vi "COM_get_data.vi"(8 "data":u8[](array[numeric]), 10 "baud rate (9600)":u32=115200 caption="波特率(115200)", 11 "VISA name":refnum<visa-resource-name>) -> (2 "data out":u8[](array[numeric]), 3 "return":i32)   [LabVIEW 2016]
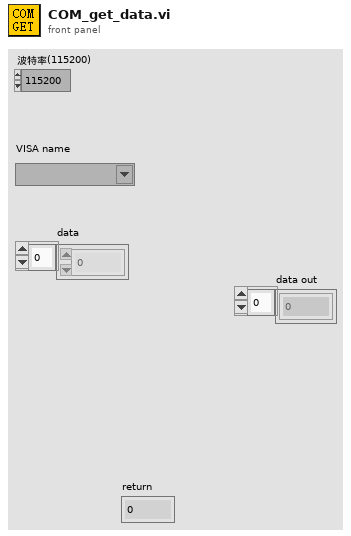
[diagram p1: front panel]
types:
  T1 = enum16{"initial", "write", "read", "release", "change"}
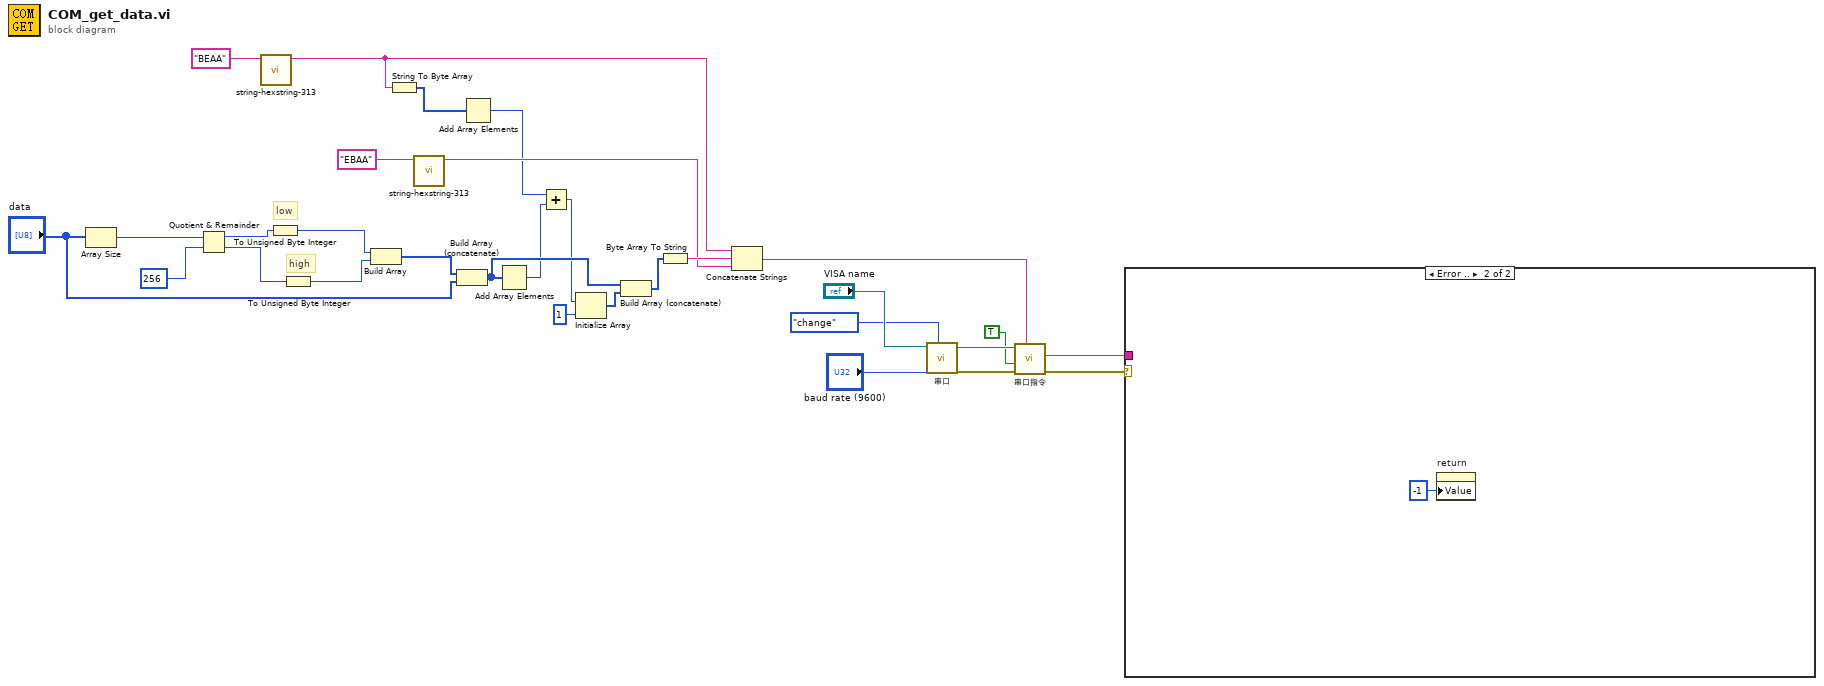
[diagram p0: block diagram]
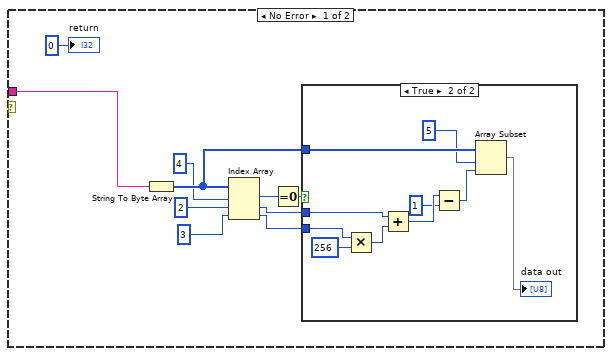
[diagram p2: hidden frame]
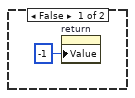
[diagram p3: hidden frame]
diagram:
  # "high"
  # "low"
  n1 = Array Size(array="data") -> (size(s)=w10:i32)
  n2 = Quotient & Remainder(x=w10, y=256) -> (x-y*floor(x/y)=w28:i32, floor(x/y)=w29:i32)
  n3 = call "string-hexstring-313.vi"("字符串"="BEAA") -> ("十六进制整型字符串"=w15:string)  [unwired: 10 in]
  n4 = To Unsigned Byte Integer(number=w28) -> (unsigned 8bit integer=w26:u8)
  n5 = To Unsigned Byte Integer(number=w29) -> (unsigned 8bit integer=w25:u8)
  n6 = Build Array(w26, w25) -> (w24:u8[])
  n7 = String To Byte Array(string=w15) -> (unsigned byte array=w14:u8[])
  n8 = call "string-hexstring-313.vi"("字符串"="EBAA") -> ("十六进制整型字符串"=w16:string)  [unwired: 10 in]
  n9 = Build Array (concatenate)(w24, "data") -> (w19:u8[])
  n10 = Add Array Elements(numeric array=w14) -> (sum=w13:u8)
  n11 = Add Array Elements(numeric array=w19) -> (sum=w12:u8)
  n12 = Add(x=w13, y=w12) -> (x+y=w11:u8)
  n13 = Initialize Array(w11, 1 ("dimension size")) -> (w20:u8[])
  n14 = Build Array (concatenate)(w19, w20) -> (w18:u8[])
  n15 = Byte Array To String(unsigned byte array=w18) -> (string=w22:string)
  n16 = Concatenate Strings(w15, w22, w16) -> (w4:string)
  n17 = call "串口.vi"("case"=T1."change", "baud rate (9600)"="baud rate (9600)", "VISA name"="VISA name") -> ("error out"=w5:errorcluster, "VISA resource name out"=w7:refnum<visa-resource-name>)  [unwired: 5 in, 2 out]
  n18 = call "串口指令.vi"("write buffer"=w4, "error in"=w5, "是否握手"=TRUE, "VISA resource name"=w7) -> ("error out"=w3:errorcluster, "outputString"=w2:string)  [unwired: 3 in, 3 out]
  n19 = case shown="Error .." w3 {
    tunnel: w2 -> [w31 _]
    frame No Error {
      n20 = String To Byte Array(string=w31) -> (unsigned byte array=w39:u8[])
      n21 = Index Array(array=w39, index #1=4 ("index"), index #2=2 ("index"), index #3=3 ("index")) -> (element #1=w36:u8, element #2=w37:u8, element #3=w38:u8)
      n22 = Equal To 0?(x=w36) -> (x = 0?=w35:bool)
      n23 = case shown="True" w35 {
        tunnel: w37 -> [_ w48]
        tunnel: w38 -> [_ w51]
        tunnel: w39 -> [_ w47]
        frame False {
          n24 = property on="return" class="DigNum (strict)"("Value"=-1 ("return")) -> ()  [unwired: 2 in, 2 out]
        }
        frame True {
          n25 = Multiply(x=w51, y=u16 256) -> (x*y=w49:u16)
          n26 = Add(x=w48, y=w49) -> (x+y=w45:u16)
          n27 = Subtract(x=w45, y=u16 1) -> (x-y=w43:u16)
          n28 = Array Subset(array=w47, index=5, length=w43) -> (→"data out":u8[])
        }
      }
      "return" <- 0 ("return")
    }
    frame Error {
      n29 = property on="return" class="DigNum (strict)"("Value"=-1 ("return")) -> ()  [unwired: 2 in, 2 out]
    }
  }
